vi "UpdatePrefFromXML.vi"(8 "error in (no error)":errorcluster, 10 "PrefItemNode in":refnum<k20>, 11 "Preferences in":refnum<class "SetListPrefs.lvclass">) -> (0 "error out":errorcluster, 1 "UpdateResult":T3, 2 "PrefItemNode out":refnum<k20>, 3 "Preferences out":refnum<class "SetListPrefs.lvclass">)   [LabVIEW 2013, in "SetListPrefs.lvclass"]
uses:
  SetListPrefs.lvclass
  UpdateResult.ctl
  PrefCluster.ctl
  <vilib>/Utility/miscctls.llb/LVRectTypeDef.ctl
  SetListPrefs.lvclass/SetListPrefs.ctl
  <vilib>/xml/Close Reference(Node).vi
  <vilib>/xml/NI_XML.lvlib
  <resource>/objmgr/DOMUserDefRef.rc
panel:
  in  "PrefCluster":T1
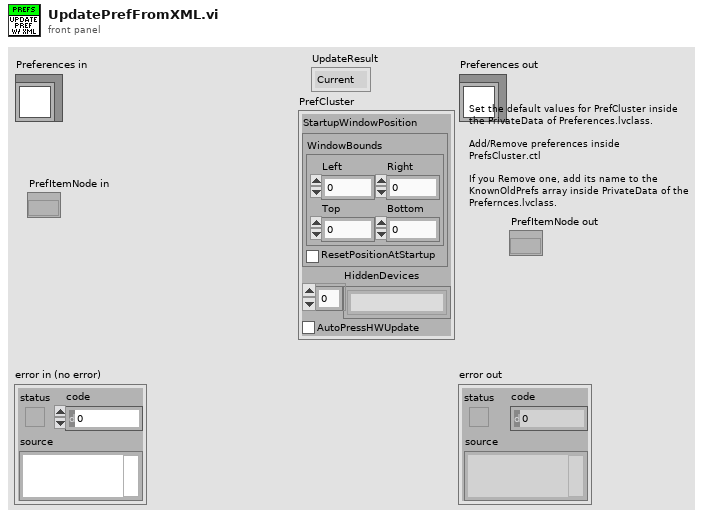
[diagram p1: front panel]
types:
  T1 = typedef "SetListPrefs.lvclass/PrefCluster.ctl" = cluster{"StartupWindowPosition":cluster{"WindowBounds":T2, "ResetPositionAtStartup":bool}, "HiddenDevices":string[], "AutoPressHWUpdate":bool}
  T2 = typedef "LVRectTypeDef.ctl" = cluster{"Left":i16, "Top":i16, "Right":i16, "Bottom":i16}
  T3 = typedef "SetListPrefs.lvclass/UpdateResult.ctl" = enum16{"Current", "Old", "Unknown"}
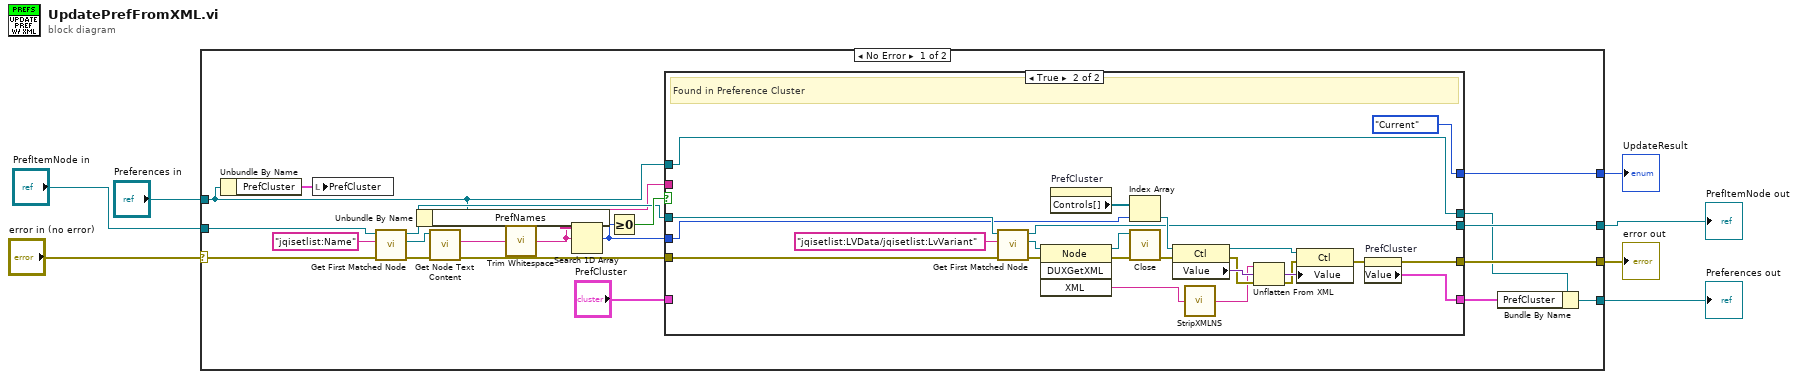
[diagram p0: block diagram]
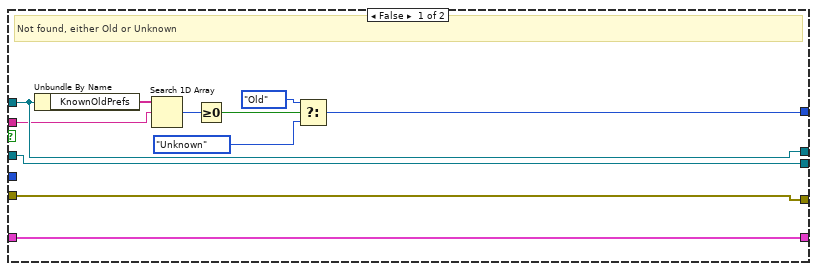
[diagram p2: hidden frame]
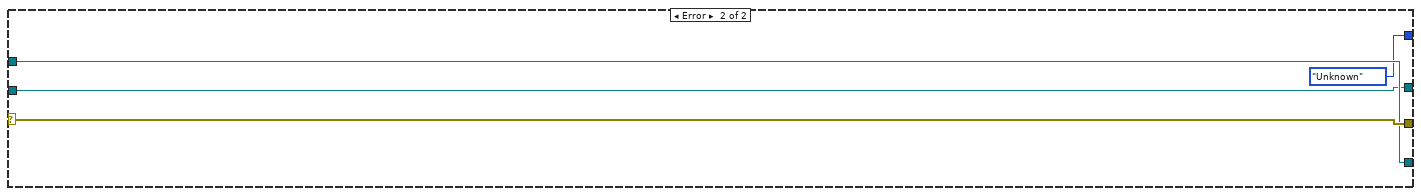
[diagram p3: hidden frame]
diagram:
  n1 = case shown="No Error" "error in (no error)" {
    selector: "error in (no error)" -> [w25 w67]
    tunnel: [w20 w67] -> w6
    tunnel: [w13 w66] -> w4
    tunnel: "Preferences in" -> [w15 w66]
    tunnel: "PrefItemNode in" -> [w27 w65]
    tunnel: [w18 w65] -> w2
    tunnel: [w28 UpdateResult."Unknown" ("UpdateResult")] -> w1
    frame No Error {
      n2 = Unbundle By Name(w15) -> ("PrefCluster"=w16:T1)
      n3 = local write "PrefCluster"(w16) -> ()
      n4 = call <vilib>:"Get First Matched Node.vi"("error in (no error)"=w25, "XPath expression"="jqisetlist:Name", "node in"=w27) -> ("error out"=w23:errorcluster, "node result"=w24:refnum<k20>, "node out"=w19:refnum<k20>)  [unwired: 6 in]
      n5 = Unbundle By Name(w15) -> ("PrefNames"=w22:string[])
      n6 = call <vilib>:"Get Node Text Content.vi"("error in (no error)"=w23, "node in"=w24) -> ("error out"=w8:errorcluster, "node text"=w10:string)  [unwired: 7 in, 1 out]
      n7 = call <vilib>:"Trim Whitespace.vi"("string"=w10) -> ("trimmed string"=w9:string)  [unwired: 1 in]
      n8 = Search 1D Array(1D array=w22, element=w9) -> (index of element=w17:i32)  [unwired: 1 in]
      n9 = Greater Or Equal To 0?(x=w17) -> (x >= 0?=w21:bool)
      n10 = case shown="True" w21 {
        tunnel: [w34 UpdateResult."Current" ("UpdateResult")] -> w28
        tunnel: w8 -> [w33 w62]
        tunnel: [w33 w43] -> w20
        tunnel: w19 -> [w32 w61]
        tunnel: [w32 w46] -> w18
        tunnel: w17 -> [_ w54]
        tunnel: w15 -> [w30 w45]
        tunnel: [w30 w45] -> w14
        tunnel: "PrefCluster" -> [w31 _]
        tunnel: [w31 w42] -> w11
        tunnel: w9 -> [w29 _]
        frame False {
          # "Not found, either Old or Unknown"
          n11 = Unbundle By Name(w30) -> ("KnownOldPrefs"=w39:string[])
          n12 = Search 1D Array(1D array=w39, element=w29) -> (index of element=w38:i32)  [unwired: 1 in]
          n13 = Greater Or Equal To 0?(x=w38) -> (x >= 0?=w37:bool)
          n14 = Select(t=UpdateResult."Old" ("UpdateResult"), s=w37, f=UpdateResult."Unknown" ("UpdateResult")) -> (s? t:f=w34:T3)
        }
        frame True {
          # "Found in Preference Cluster"
          n15 = call <vilib>:"Get First Matched Node.vi"("error in (no error)"=w62, "XPath expression"="jqisetlist:LVData/jqisetlist:LvVariant", "node in"=w61) -> ("error out"=w58:errorcluster, "node result"=w59:refnum<k20>, "node out"=w46:refnum<k20>)  [unwired: 6 in]
          n16 = invoke class="Node" method="DUXGetXML"(reference=w59, error in=w58) -> (reference out=w57:refnum<k20>, error out=w56:errorcluster, "XML"=w41:string)  [unwired: 2 in, 1 out]
          n17 = property on="PrefCluster" class="Clust (strict)"() -> ("Controls[]"=w55:refnum<vi>[])  [unwired: 2 in, 2 out]
          n18 = Index Array(array=w55, index=w54) -> (element=w53:refnum<vi>)
          n19 = call-poly <vilib>:"Close.vi"("error in (no error)"=w56, "node"=w57) -> ("error out"=w52:errorcluster)  [unwired: 7 in]
          n20 = property class="Ctl"(reference=w53, error in=w52) -> (reference out=w47:refnum<vi>, error out=w50:errorcluster, "Value"=w51:variant)
          n21 = call "StripXMLNS.vi"("XML in"=w41) -> ("XML out"=w40:string)
          n22 = Unflatten From XML(xml string=w40, type=w51, error in (no error)=w50) -> (value=w49:variant, error out=w48:errorcluster)
          n23 = property class="Ctl"(reference=w47, error in=w48, "Value"=w49) -> (error out=w44:errorcluster)  [unwired: 1 out]
          n24 = property on="PrefCluster" class="Clust (strict)"(error in=w44) -> (error out=w43:errorcluster, "Value"=w42:T1)  [unwired: 1 in, 1 out]
        }
      }
      n25 = Bundle By Name(cluster=w14, "PrefCluster"=w11) -> (w13:refnum<class "SetListPrefs.lvclass">)
    }
    frame Error {
    }
  }
  "error out" <- w6
  "Preferences out" <- w4
  "PrefItemNode out" <- w2
  "UpdateResult" <- w1
